vi "test Create Custom Anchor.vi"(8 "error in (no error)":errorcluster, 11 "TestCase in":refnum<class "AnchorTests.lvclass">) -> (0 "error out":errorcluster, 3 "TestCase out":refnum<class "AnchorTests.lvclass">)   [LabVIEW 2014, in "AnchorTests.lvclass"]
uses:
  AnchorTests.lvclass
  <vilib>/addons/_JKI Toolkits/VI Tester/TestCase.llb/TestCase.lvclass
  SPLAT/Anchor/Anchor.lvclass
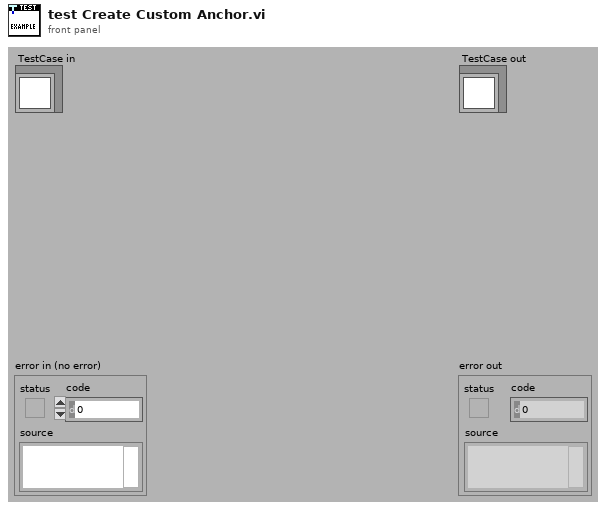
[diagram p1: front panel]
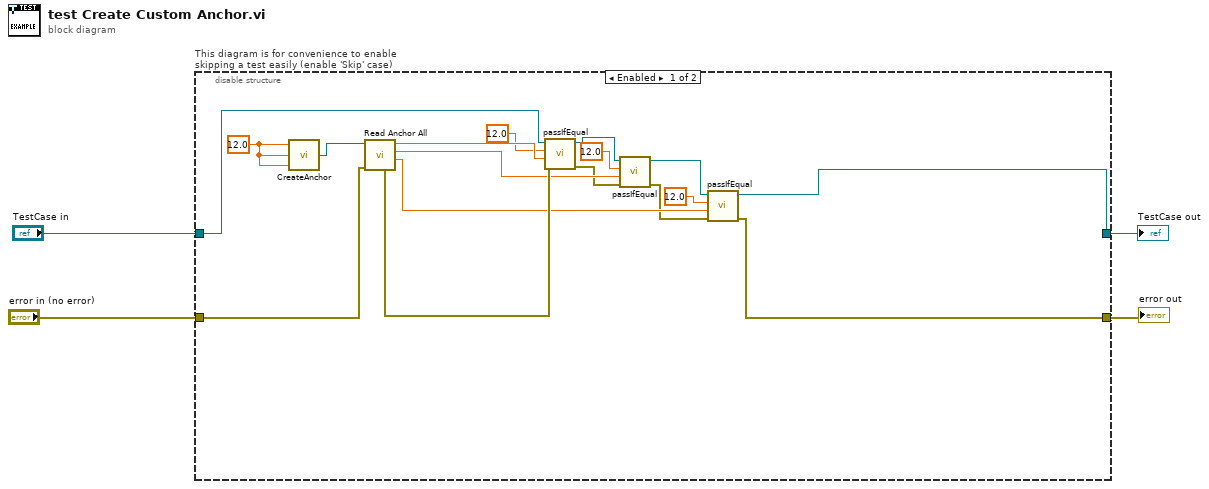
[diagram p0: block diagram]
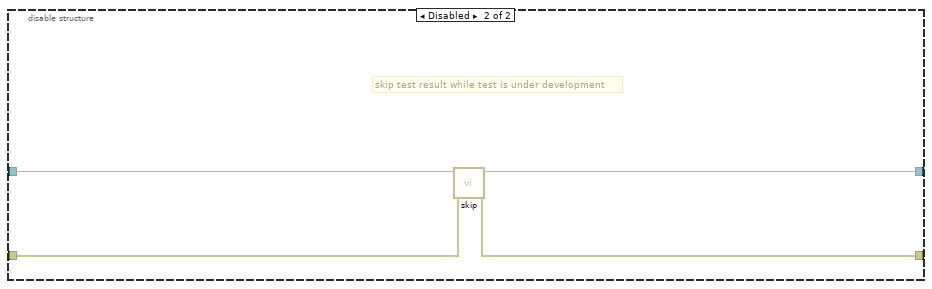
[diagram p2: hidden frame]
diagram:
  n1 = disable-structure "This diagram is for convenience to enable skipping a test easily (enable 'Skip' case)" shown="Enabled" {
    disable-tunnel: "TestCase in" -> [w17 w25]
    disable-tunnel: [w8 w23] -> w1
    disable-tunnel: [w7 w24] -> w3
    disable-tunnel: "error in (no error)" -> [w19 w22]
    frame Enabled {
      w21 = 12.0 ("Anchor ID")
      n2 = call "CreateAnchor.vi"("Anchor Y"=w21, "Anchor X"=w21, "Anchor ID"=w21) -> ("Anchor Out"=w20:refnum<class "Anchor.lvclass">)
      n3 = call "Read Anchor All.vi"("error in (no error)"=w19, "Anchor in"=w20) -> ("AnchorY"=w14:dbl, "AnchorX"=w15:dbl, "AnchorID"=w16:dbl, "error out"=w18:errorcluster)  [unwired: 4 in, 2 out]
      n4 = call-dynamic "passIfEqual.vi"("error in (no error)"=w18, "y"=w16, "x"=12.0 ("Anchor ID"), "TestCase in"=w17) -> ("error out"=w5:errorcluster, "TestCase out"=w10:refnum<class "AnchorTests.lvclass">)  [unwired: 6 in]
      n5 = call-dynamic "passIfEqual.vi"("error in (no error)"=w5, "y"=w15, "x"=12.0 ("Anchor ID"), "TestCase in"=w10) -> ("error out"=w6:errorcluster, "TestCase out"=w9:refnum<class "AnchorTests.lvclass">)  [unwired: 6 in]
      n6 = call-dynamic "passIfEqual.vi"("error in (no error)"=w6, "y"=w14, "x"=12.0 ("Anchor ID"), "TestCase in"=w9) -> ("error out"=w7:errorcluster, "TestCase out"=w8:refnum<class "AnchorTests.lvclass">)  [unwired: 6 in]
    }
    frame Disabled {
      # "skip test result while test is under development"
      n7 = call <vilib>:"skip.vi"("error in (no error)"=w22, "TestCase in"=w25) -> ("error out"=w24:errorcluster, "TestCase out"=w23:refnum<class "AnchorTests.lvclass">)  [unwired: 8 in]
    }
  }
  "error out" <- w3
  "TestCase out" <- w1
